vi "foodassert.vi"(8 "价格(小于等于） 2":dbl, 9 "名称 2":string, 10 "价格":dbl, 11 "食品名称":string) -> (1 "正确":bool, 2 "价格(小于等于） 3":dbl, 3 "名称 3":string)   [LabVIEW 2013, in "FoodBase.lvclass"]
uses:
  FoodBase.lvclass
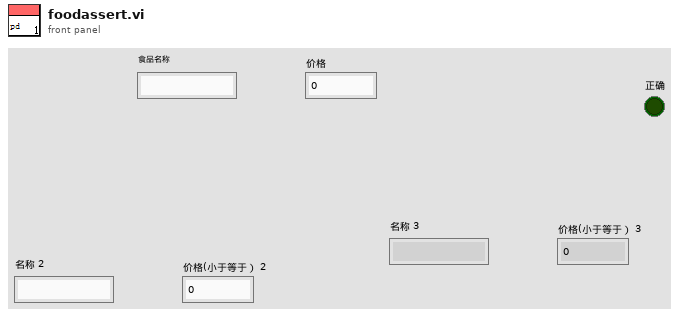
[diagram p1: front panel]
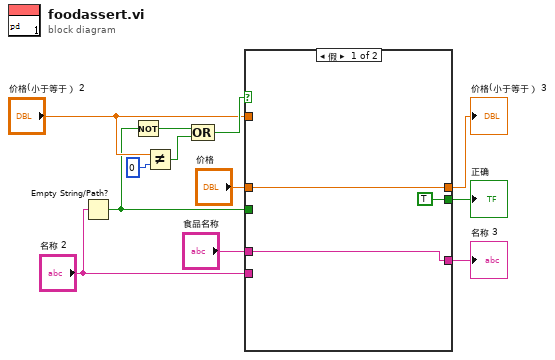
[diagram p0: block diagram]
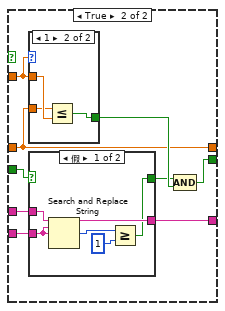
[diagram p2: hidden frame]
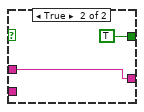
[diagram p3: hidden frame]
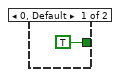
[diagram p4: hidden frame]
diagram:
  n1 = Empty String/Path?(string/path="名称 2") -> (empty?=w1:bool)
  n2 = Not(x=w1) -> (.not. x?=w2:bool)
  n3 = Not Equal?(x="价格(小于等于） 2", y=0) -> (x != y?=w11:bool)
  n4 = Compound Arithmetic op=OR(w2, w11) -> (w10:bool)
  n5 = case shown="假" w10 {
    tunnel: "食品名称" -> [w15 w18]
    tunnel: "价格" -> [w14 w23]
    tunnel: [w15 w16] -> w7
    tunnel: [w14 w23] -> w6
    tunnel: [TRUE w21] -> w5
    tunnel: "名称 2" -> [_ w17]
    tunnel: "价格(小于等于） 2" -> [_ w22]
    tunnel: w1 -> [_ w20]
    frame False {
    }
    frame True {
      n6 = case shown="1" w22 {
        tunnel: w22 -> [_ w36]
        tunnel: [TRUE w35] -> w24
        tunnel: w23 -> [_ w34]
        frame 0, Default {
        }
        frame 1 {
          n7 = Less Or Equal?(x=w34, y=w36) -> (x <= y?=w35:bool)
        }
      }
      n8 = case shown="假" w20 {
        tunnel: [w25 TRUE] -> w19
        tunnel: w18 -> [w30 w31]
        tunnel: w17 -> [w29 _]
        tunnel: [w28 w31] -> w16
        frame False {
          n9 = Search and Replace String(input string=w30, search string=w29, replace string=w29) -> (result string=w28:string, number of replacements=w27:i32)  [unwired: 5 in, 2 out]
          n10 = Greater Or Equal?(x=w27, y=1) -> (x >= y?=w25:bool)
        }
        frame True {
        }
      }
      n11 = Compound Arithmetic op=AND(w19, w24) -> (w21:bool)
    }
  }
  "名称 3" <- w7
  "价格(小于等于） 3" <- w6
  "正确" <- w5
